vi "GetCurrentSong.vi"(0 "reference in":refnum<class "MusicPlayer.lvclass">, 11 "Error In":errorcluster) -> (4 "reference out":refnum<class "MusicPlayer.lvclass">, 8 "Song Path":path, 10 "Song Name":string, 15 "Error Out":errorcluster)   [LabVIEW 2022 SP3, in "MusicPlayer.lvclass"]
uses:
  MusicPlayer.lvclass
  MusicPlayer.lvclass/MusicPlayer.ctl
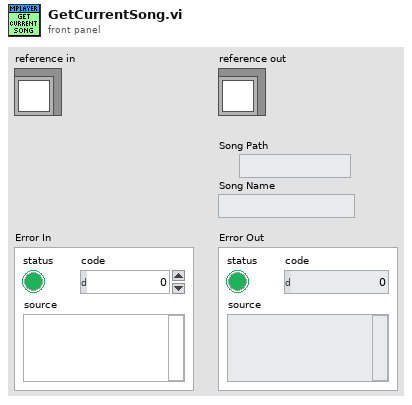
[diagram p1: front panel]
types:
  T1 = typedef "MusicPlayer.lvclass/ObjectAttributes.ctl" = cluster{"MediaPlayer":refnum<k7>, "Playlist":path[], "Index":u32}
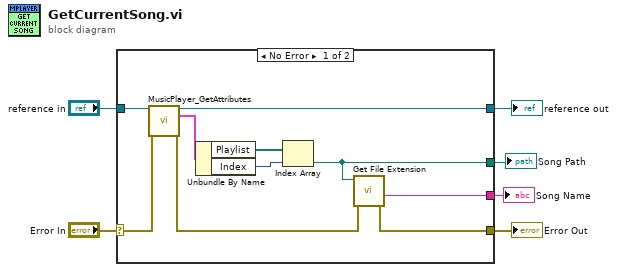
[diagram p0: block diagram]
diagram:
  n1 = case shown="No Error" "Error In" {
    selector: "Error In" -> [w16 w18]
    tunnel: [w7 w18] -> w5
    tunnel: [w13 w17] -> w3
    tunnel: "reference in" -> [w14 w17]
    tunnel: [w10 _] -> w2
    tunnel: [w9 _] -> w1
    frame No Error {
      n2 = call "MusicPlayer_GetAttributes.vi"("reference in"=w14, "error in (no error)"=w16) -> ("reference out"=w13:refnum<class "MusicPlayer.lvclass">, "Data"=w15:T1, "error out"=w8:errorcluster)  [unwired: 10 in, 1 out]
      n3 = Unbundle By Name(w15) -> ("Playlist"=w12:path[], "Index"=w11:u32)
      n4 = Index Array(array=w12, index=w11) -> (element=w10:path)
      n5 = call <vilib>:"Get File Extension.vi"("error in (no error)"=w8, "file"=w10) -> ("error out"=w7:errorcluster, "filename without extension"=w9:string)  [unwired: 5 in, 3 out]
    }
    frame Error {
    }
  }
  "Error Out" <- w5
  "reference out" <- w3
  "Song Path" <- w2
  "Song Name" <- w1
